vi "Mode_Ref_API.vi"(0 "DVR In":refnum<data-value>, 11 "Error In":errorcluster) -> (4 "DVR Out":refnum<data-value>, 6 "VI Ref":refnum<vi>, 8 "Mode Ref":refnum<vi>, 15 "Error out":errorcluster)   [LabVIEW 2020, in "Test.lvclass"]
doc: "Mode Reference API"
uses:
  Test.lvclass
  Children/INL DNL Test/INL DNL Test.lvclass
  Test.lvclass/Test.ctl
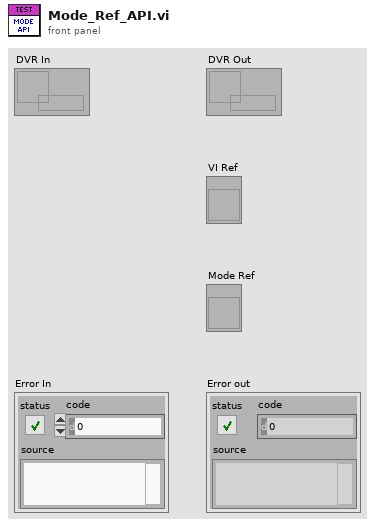
[diagram p1: front panel]
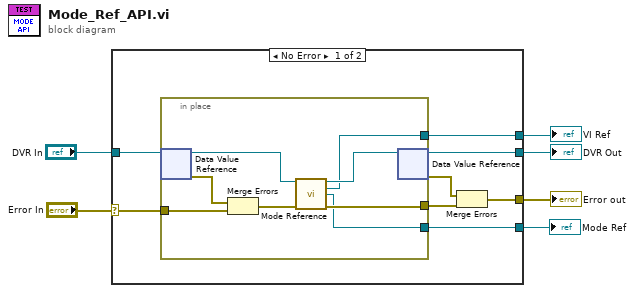
[diagram p0: block diagram]
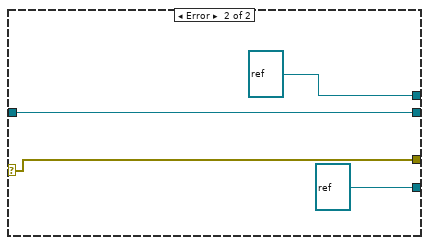
[diagram p2: hidden frame]
diagram:
  n1 = case shown="No Error" "Error In" {
    selector: "Error In" -> [w14 w24]
    tunnel: "DVR In" -> [w13 w25]
    tunnel: [w12 w25] -> w4
    tunnel: [w8 w24] -> w3
    tunnel: [w11 refnum<vi> refnum ("VI Refnum")] -> w2
    tunnel: [w7 refnum<vi> refnum ("Mode Ref")] -> w1
    frame No Error {
      n2 = in-place {
        in-place-border: w14 -> [w22]
        in-place-border: [w18] -> w10
        in-place-border: [w16] -> w11
        in-place-border: [w15] -> w7
        n3 = in-place-dvr #1(w13) -> (w19:refnum<class "Test.lvclass">, w21:errorcluster)
        n4 = Merge Errors(w21, w22) -> (w20:errorcluster)
        n5 = call-dynamic "Mode Reference.vi"("Test in"=w19, "Error in"=w20) -> ("Test out"=w17:refnum<class "Test.lvclass">, "VI Refnum"=w16:refnum<vi>, "Mode Ref"=w15:refnum<vi>, "Error out"=w18:errorcluster)  [unwired: 10 in]
        n6 = in-place-dvr #1(w17) -> (w12:refnum<data-value>, w9:errorcluster)
      }
      n7 = Merge Errors(w9, w10) -> (w8:errorcluster)
    }
    frame Error {
    }
  }
  "DVR Out" <- w4
  "Error out" <- w3
  "VI Ref" <- w2
  "Mode Ref" <- w1
